vi "AbsI16.vi"(4 "x":i16) -> (1 "Abs(x)":i16, 2 "Overflow?":bool)   [LabVIEW 2017, in "GPOverflow.lvlib"]
doc: "Returns the absolute value of <B>x</B> keeping track of numeric overflow.\n\n<B>Overflow?</B> will be True if overflow occurred. The output will saturate in case of overflow.\n\nThis VI is inlined.\n\nSteen Schmidt\nGPower\n26/12 2013"
uses:
  GPOverflow.lvlib
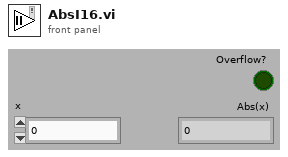
[diagram p1: front panel]
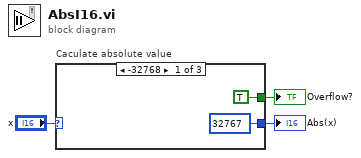
[diagram p0: block diagram]
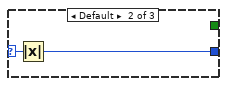
[diagram p2: hidden frame]
diagram:
  n1 = case "Caculate absolute value" shown="-32768" "x" {
    selector: "x" -> [_ w7 w8]
    tunnel: [i16 32767 w6 w8] -> w2
    tunnel: [TRUE _ _] -> w1
    frame -32768 {
    }
    frame Default {
      n2 = Absolute Value(x=w7) -> (abs(x)=w6:i16)
    }
    frame 0.. {
    }
  }
  "Abs(x)" <- w2
  "Overflow?" <- w1
